vi "CalcArea.vi"(8 "Error In":errorcluster, 11 "Rectangle in":refnum<class "Rectangle.lvclass">) -> (0 "Error Out":errorcluster, 2 "Area":dbl, 3 "Rectangle out":refnum<class "Rectangle.lvclass">)   [LabVIEW 2021, in "Rectangle.lvclass"]
doc: "Calc a area of rectangle object."
uses:
  Rectangle.lvclass
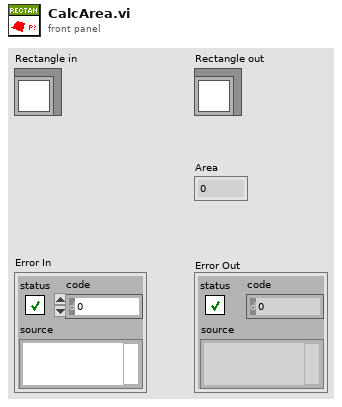
[diagram p1: front panel]
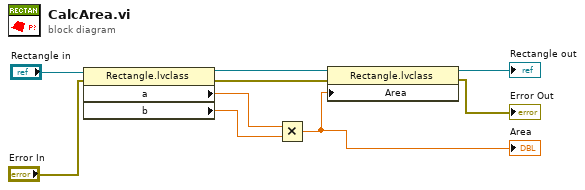
[diagram p0: block diagram]
diagram:
  n1 = property class="Rectangle.lvclass"(reference="Rectangle in", error in="Error In") -> (reference out=w7:refnum<class "Rectangle.lvclass">, error out=w6:errorcluster, "a"=w5:dbl, "b"=w4:dbl)
  n2 = Multiply(x=w5, y=w4) -> (x*y=w3:dbl)
  "Area" <- w3
  n3 = property class="Rectangle.lvclass"(reference=w7, error in=w6, "Area"=w3) -> (reference out=→"Rectangle out":refnum<class "Rectangle.lvclass">, error out=→"Error Out":errorcluster)
